vi "DataCNT-New.vi"(8 "error in (no error)":errorcluster) -> (0 "error out":errorcluster, 3 "DataCNT out":T1)   [LabVIEW 2017, in "Data Container.lvlib"]
uses:
  Data Container.lvlib
  TypeDef/Def-DataCNT.ctl
  TypeDef/Def-DataCNT Ico.ctl
panel:
  # "Connector Pane"
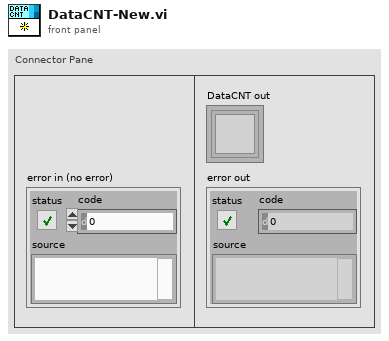
[diagram p1: front panel]
types:
  T1 = typedef "Data Container.lvlib/Def-DataCNT.ctl" = refnum<k1>
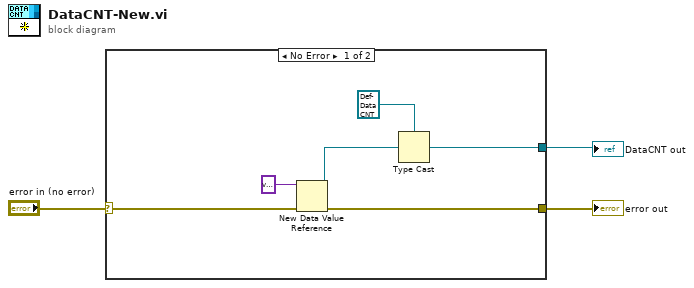
[diagram p0: block diagram]
diagram:
  n1 = case shown="No Error" "error in (no error)" {
    selector: "error in (no error)" -> [w9 w10]
    tunnel: [w7 w10] -> w2
    tunnel: [w5 _] -> w1
    frame No Error {
      n2 = New Data Value Reference(data value=variant, error in=w9) -> (data value reference=w6:refnum<data-value>, error out=w7:errorcluster)
      n3 = Type Cast(type=T1 refnum ("Container"), x=w6) -> (*(type *) &x=w5:T1)
    }
    frame Error {
    }
  }
  "error out" <- w2
  "DataCNT out" <- w1
